vi "MoveStepCommand.vi"(8 "error in (no error)":errorcluster, 10 "MultiCVT":bool, 11 "Tapedrive_ESP301 in":refnum<class "Tapedrive_ESP301.lvclass">) -> (0 "error out":errorcluster, 2 "String":string, 3 "Tapedrive_ESP301.lvclass":refnum<class "Tapedrive_ESP301.lvclass">)   [LabVIEW 2013, in "Tapedrive_ESP301.lvclass"]
uses:
  Tapedrive_ESP301.lvclass
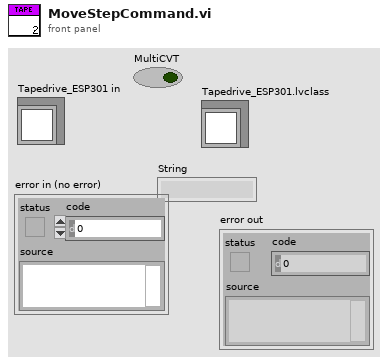
[diagram p1: front panel]
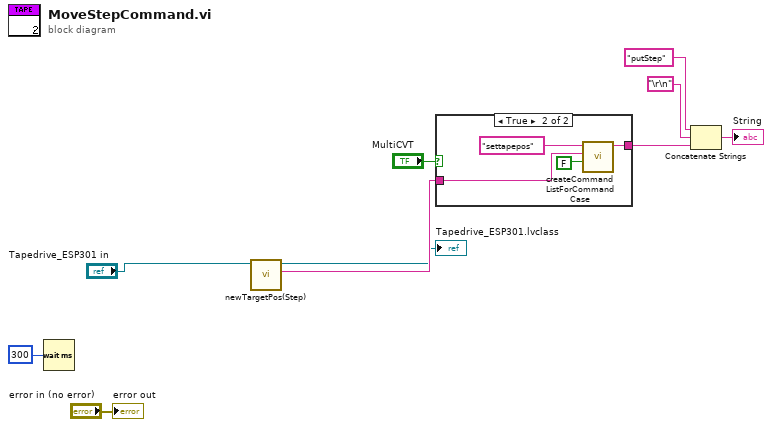
[diagram p0: block diagram]
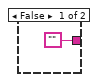
[diagram p2: hidden frame]
diagram:
  n1 = Wait (ms)(milliseconds to wait=u32 300) -> ()  [unwired: 1 out]
  n2 = call "newTargetPos(Step).vi"("Tapedrive_ESP301 in"="Tapedrive_ESP301 in") -> ("String"=w10:string, "Tapedrive_ESP301 out"=→"Tapedrive_ESP301.lvclass":refnum<class "Tapedrive_ESP301.lvclass">)  [unwired: 9 in]
  n3 = case shown="True" "MultiCVT" {
    tunnel: w10 -> [_ w15]
    tunnel: ["" w12] -> w3
    frame False {
    }
    frame True {
      n4 = call "createCommandListForCommandCase.vi"("immediate Check (only once)"=FALSE, "setvalue"=w15, "command"="settapepos") -> ("new commands"=w12:string)  [unwired: 8 in]
    }
  }
  n5 = Concatenate Strings("putStep" ("string"), "\r\n", w3) -> (→"String":string)
  "error out" <- "error in (no error)"
